vi "(auto) Count balls (SubVI).vi"(11 "Circles Calibrated (Shape Detection 1)":T1(array[cluster])) -> (3 "balls counter":i32)   [LabVIEW 2017]
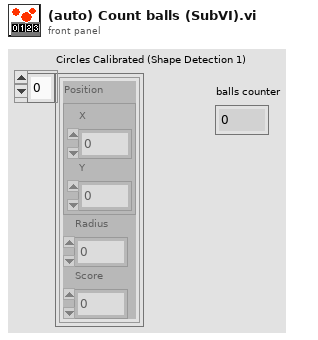
[diagram p1: front panel]
types:
  T1 = cluster{"Position":cluster{"X":sgl, "Y":sgl}, "Radius":dbl, "Score":dbl}[]
  T2 = cluster{"Position":cluster{"X":sgl, "Y":sgl}, "Radius":dbl, "Score":dbl}
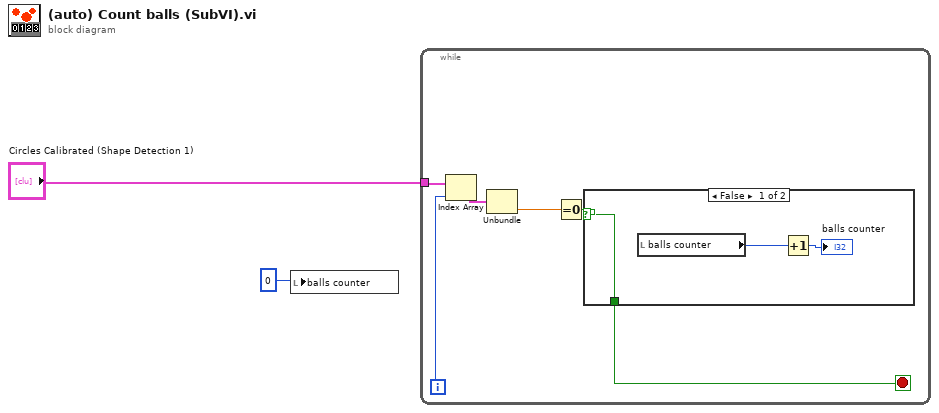
[diagram p0: block diagram]
diagram:
  n1 = local write "balls counter"(0 ("balls counter")) -> ()
  n2 = while {
    tunnel: "Circles Calibrated (Shape Detection 1)" -> [w8]
    i -> [w7]
    stop <- w3 stop-if-true
    n3 = Index Array(array=w8, index=w7) -> (element=w6:T2)
    n4 = Unbundle(w6) -> ("Score"=w5:dbl)  [unwired: 2 out]
    n5 = Equal To 0?(x=w5) -> (x = 0?=w4:bool)
    n6 = case shown="False" w4 {
      selector: w4 -> [w11 w12]
      tunnel: [w11 w12] -> w3
      frame False {
        n7 = local read "balls counter"() -> (w10:i32)
        n8 = Increment(x=w10) -> (x+1=→"balls counter":i32)
      }
      frame True {
      }
    }
  }
